vi "LOWER CASE AND UPPER CASE CONVERSION.vi"() -> ()   [LabVIEW 2019]
panel:
  out "LOWER CASE OUTPUT":string
  out "UPPER CASE OUTPUT":string
  in  "INPUT STRING":string="coimbatore"
  # "LOWER CASE AND UPPER CASE CONVERSION"
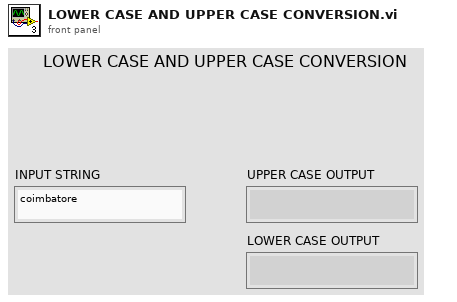
[diagram p1: front panel]
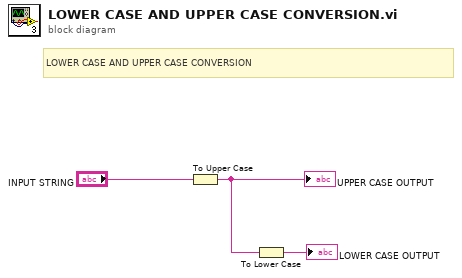
[diagram p0: block diagram]
diagram:
  # "LOWER CASE AND UPPER CASE CONVERSION"
  n1 = To Upper Case(1:"INPUT STRING") -> (0:w2:string)
  "UPPER CASE OUTPUT" <- w2
  n2 = To Lower Case(string=w2) -> (all lower case string=→"LOWER CASE OUTPUT":string)
